vi "CVT String StaticRead.vi"(3 "error in (no error)":errorcluster, 5 "Tag Name":string) -> (0 "error out":errorcluster, 1 "Value":string)   [LabVIEW 2020, in "Current Value Table(Rebuild).lvlib"]
uses:
  Current Value Table(Rebuild).lvlib
  DataTypes/String_Static Read.vi
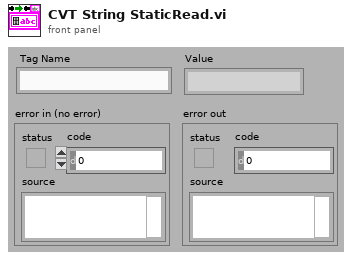
[diagram p1: front panel]
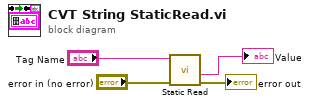
[diagram p0: block diagram]
diagram:
  n1 = call-poly "Static Read.vi"("error in (no error)"="error in (no error)", "Tag Name"="Tag Name") -> ("error out"=→"error out":errorcluster, "Value"=→"Value":string)  [unwired: 8 in]
